vi "Simulation Robot Open.vi"(8 "error in (no error)":errorcluster, 11 "RoboSimIDs":T1) -> (0 "error out":errorcluster, 2 "initial position":sgl[](array[numeric]), 3 "Robot":T3)   [LabVIEW 2015]
doc: "Begins a simulation of the Cal Climber."
uses:
  Multi Bot Code/RobotData.ctl
  <instrlib>/DC Motor Controller/HAIOL/DC Motor Controller.lvclass
  Multi Bot Code/SensorType.ctl
  SimulationIDs.ctl
  <vilib>/robotics/Simulator/Engine/ctl/DeviceID.ctl
  <vilib>/robotics/Simulator/Interface/Simulator References/Get Robot Body Reference.vi
  <vilib>/robotics/Simulator/Interface/Simulator References/Get Sensor Reference.vi
  <vilib>/robotics/Simulator/NI_Robotics_Simulator.lvlib
  <resource>/objmgr/LVODE.rc
  <instrlib>/DC Motor Controller/HAIOL/Simulator/DC Motor Controller Simulator.lvclass
panel:
  out "sorted array":string[](array[string])
  out "SensorType":T2 items=["BumperSensor"=1, "DistanceSensor"=2, "AccelerometerSensor"=3, "Wall Sensor"=4, "Unknown"=0]
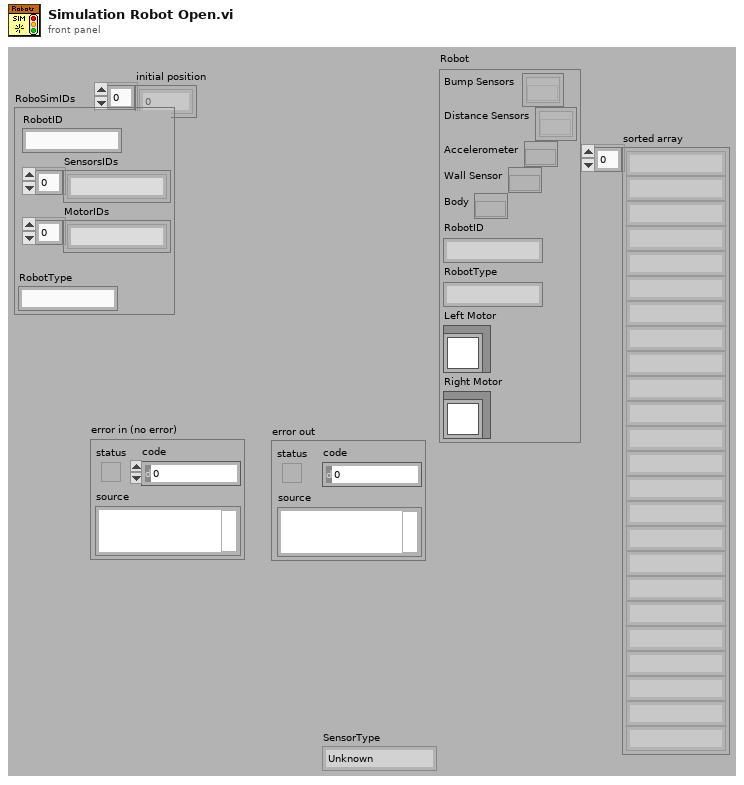
[diagram p1: front panel]
types:
  T1 = typedef "SimulationIDs.ctl" = cluster{"RobotID":string, "SensorsIDs":string[], "MotorIDs":string[], "RobotType":string}
  T2 = typedef "SensorType.ctl" = u16
  T3 = typedef "RobotData.ctl" = cluster{"Bump Sensors":refnum<k20>[], "Distance Sensors":refnum<k20>[], "Accelerometer":refnum<k20>, "Wall Sensor":refnum<k20>, "Body":refnum<k20>, "RobotID":string, "RobotType":string, "Left Motor":refnum<class "DC Motor Controller.lvclass">, "Right Motor":refnum<class "DC Motor Controller.lvclass">}
  T4 = typedef "NI_Robotics_Simulator.lvlib/DeviceID.ctl" = cluster{"robot ID":string, "sensor/actuator ID":string}
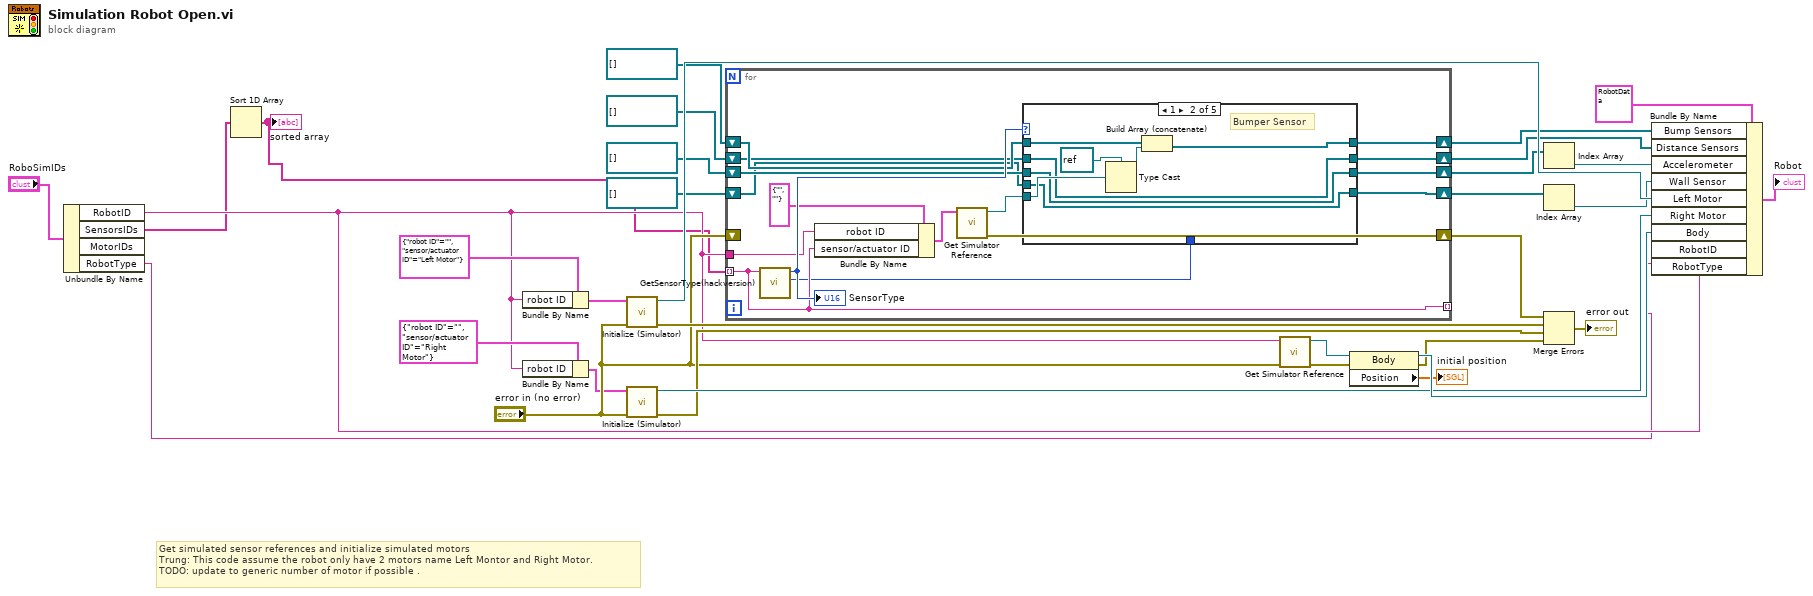
[diagram p0: block diagram]
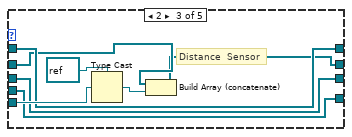
[diagram p3: hidden frame]
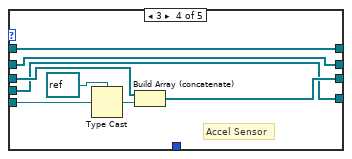
[diagram p4: hidden frame]
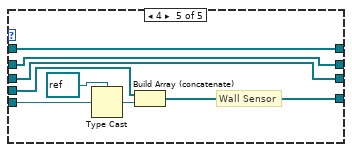
[diagram p5: hidden frame]
diagram:
  # "Get simulated sensor references and initialize simulated motors\nTrung: This code assume the robot only have 2 motors name Left Montor and Right Motor.\nTODO: update to generic number of motor if possible ."
  n1 = Unbundle By Name("RoboSimIDs") -> ("RobotID"=w4:string, "SensorsIDs"=w2:string[], "RobotType"=w3:string)  [unwired: 1 out]
  n2 = Sort 1D Array(array=w2) -> (sorted array=w1:string[])
  "sorted array" <- w1
  n3 = Bundle By Name(cluster=T4 {"robot ID"="", "sensor/actuator ID"="Left Motor"} ("Device ID"), "robot ID"=w4) -> (w21:T4)
  n4 = Bundle By Name(cluster=T4 {"robot ID"="", "sensor/actuator ID"="Right Motor"} ("Device ID"), "robot ID"=w4) -> (w5:T4)
  n5 = call <instrlib>:"Initialize (Simulator).vi"("error in (no error)"="error in (no error)", "Device ID"=w21) -> ("error out"=w29:errorcluster, "DC Motor Controller out"=w30:refnum<class "DC Motor Controller.lvclass">)  [unwired: 8 in]
  n6 = call <instrlib>:"Initialize (Simulator).vi"("error in (no error)"="error in (no error)", "Device ID"=w5) -> ("error out"=w27:errorcluster, "DC Motor Controller out"=w28:refnum<class "DC Motor Controller.lvclass">)  [unwired: 8 in]
  n7 = for {
    shift-right: [w47] -> w10
    shift-left: refnum<k20>[] [] ("Bump Sensors") -> [w48]
    shift-right: [w45] -> w9
    shift-left: refnum<k20>[] [] ("Distance Sensors") -> [w46]
    shift-right: [w43] -> w12
    shift-left: refnum<k20>[] [] ("Bump Sensors") -> [w44]
    shift-right: [w41] -> w14
    shift-left: refnum<k20>[] [] ("Bump Sensors") -> [w42]
    tunnel: [w35] -> _ mode=indexing
    tunnel: w1 -> [w35] mode=indexing
    tunnel: w4 -> [w40]
    shift-right: [w36] -> w7
    shift-left: "error in (no error)" -> [_]
    n8 = call "GetSensorType(hackversion).vi"("Accessors:ID"=w35) -> ("offset"=w34:i32, "SensorType"=w49:T2)  [unwired: 9 in]
    "SensorType" <- w49
    n9 = Bundle By Name(cluster=T4 {"robot ID"="", "sensor/actuator ID"=""} ("Device ID"), "robot ID"=w40, "sensor/actuator ID"=w35) -> (w39:T4)
    n10 = call-poly <vilib>:"Get Simulator Reference.vi"("device ID"=w39) -> ("error out"=w36:errorcluster, "sensor ref"=w37:refnum<k20>)  [unwired: 9 in]
    n11 = case shown="1" w49 {
      tunnel: w37 -> [_ w60 w68 w76 w84]
      tunnel: [w53 w55 w67 w75 w83] -> w47
      tunnel: w48 -> [w53 w56 w67 w75 w83]
      tunnel: [w52 w59 w62 w74 w82] -> w45
      tunnel: w46 -> [w52 w59 w64 w74 w82]
      tunnel: [w51 w58 w66 w71 w78] -> w43
      tunnel: w44 -> [w51 w58 w66 w73 w78]
      tunnel: w42 -> [w50 w57 w65 w70 w80]
      tunnel: [w50 w57 w65 w70 w79] -> w41
      tunnel: w34 -> [_ _ _ _ _]
      frame 0, Default {
      }
      frame 1 {
        # "Bumper Sensor"
        n12 = Type Cast(type=refnum<k20> refnum ("LVODE Refnum"), x=w60) -> (*(type *) &x=w54:refnum<k20>)
        n13 = Build Array (concatenate)(w56, w54) -> (w55:refnum<k20>[])
      }
      frame 2 {
        # "Distance  Sensor"
        n14 = Type Cast(type=refnum<k20> refnum ("LVODE Refnum"), x=w68) -> (*(type *) &x=w63:refnum<k20>)
        n15 = Build Array (concatenate)(w64, w63) -> (w62:refnum<k20>[])
      }
      frame 3 {
        # "Accel Sensor"
        n16 = Type Cast(type=refnum<k20> refnum ("LVODE Refnum"), x=w76) -> (*(type *) &x=w72:refnum<k20>)
        n17 = Build Array (concatenate)(w73, w72) -> (w71:refnum<k20>[])
      }
      frame 4 {
        # "Wall Sensor"
        n18 = Type Cast(type=refnum<k20> refnum ("LVODE Refnum"), x=w84) -> (*(type *) &x=w81:refnum<k20>)
        n19 = Build Array (concatenate)(w80, w81) -> (w79:refnum<k20>[])
      }
    }
  }
  n20 = call-poly <vilib>:"Get Simulator Reference.vi"("error in (no error)"="error in (no error)", "robot ID"=w4) -> ("error out"=w25:errorcluster, "robot body ref"=w26:refnum<k20>)  [unwired: 8 in]
  n21 = property class="Body"(reference=w26, error in=w25) -> (reference out=w33:refnum<k20>, error out=w24:errorcluster, "Position"=→"initial position":sgl[])
  n22 = Index Array(array=w12) -> (element=w11:refnum<k20>)  [unwired: 1 in]
  n23 = Index Array(array=w14) -> (element=w13:refnum<k20>)  [unwired: 1 in]
  n24 = Merge Errors(w7, w29, w27, w24) -> (→"error out":errorcluster)
  n25 = Bundle By Name(cluster=T3 {"Bump Sensors"=[], "Distance Sensors"=[], "Accelerometer"=refnum, "Wall Sensor"=refnum, "Body"=refnum, "RobotID"="", "RobotType"="", "Left Motor"=refnum, "Right Motor"=refnum} ("Robot"), "Bump Sensors"=w10, "Distance Sensors"=w9, "Accelerometer"=w11, "Wall Sensor"=w13, "Left Motor"=w30, "Right Motor"=w28, "Body"=w33, "RobotID"=w4, "RobotType"=w3) -> (→"Robot":T3)
